vi "Configure.vi"(7 "Manual Range (1.0 V)":dbl=1.0 format="%_3g", 8 "error in (no error)":errorcluster, 9 "Manual Resolution (0: 3.5 digits)":enum16{"3.5", "4.5", "5.5", "6.5"}(ring), 10 "Function (0: DC Volts)":u16(ring) items=["DC Volts", "AC Volts"], 11 "VISA resource name":refnum<visa-resource-name>) -> (0 "error out":errorcluster, 3 "VISA resource name out":refnum<visa-resource-name>)   [LabVIEW 2019, in "K2002.lvlib"]
uses:
  K2002.lvlib
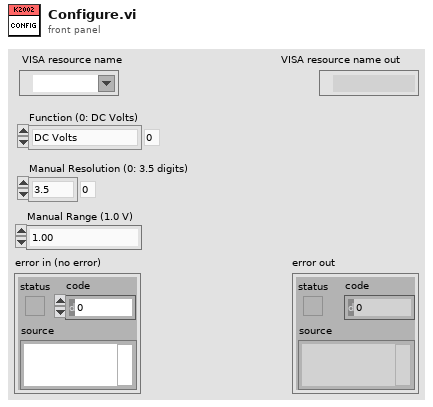
[diagram p1: front panel]
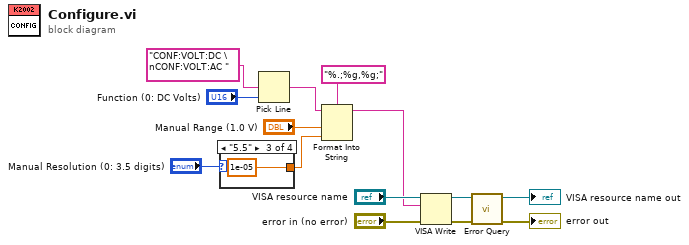
[diagram p0: block diagram]
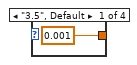
[diagram p2: hidden frame]
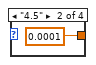
[diagram p3: hidden frame]
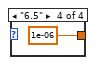
[diagram p4: hidden frame]
diagram:
  n1 = case shown="\"5.5\"" "Manual Resolution (0: 3.5 digits)" {
    tunnel: [0.001 0.0001 1e-05 1e-06] -> w1
    frame "3.5", Default {
    }
    frame "4.5" {
    }
    frame "5.5" {
    }
    frame "6.5" {
    }
  }
  n2 = Pick Line(multi-line string="CONF:VOLT:DC \nCONF:VOLT:AC " ("Function"), line index="Function (0: DC Volts)") -> (output string=w5:string)  [unwired: 1 in]
  n3 = Format Into String(format string="%.;%g,%g;", initial string=w5, "Manual Range (1.0 V)", w1) -> (resulting string=w3:string)  [unwired: 1 in, 1 out]
  n4 = VISA Write(VISA resource name="VISA resource name", write buffer=w3, error in (no error)="error in (no error)") -> (VISA resource name out=w9:refnum<visa-resource-name>, error out=w8:errorcluster)  [unwired: 1 out]
  n5 = call "Error Query.vi"("error in (no error)"=w8, "VISA resource name"=w9) -> ("error out"=→"error out":errorcluster, "VISA resource name out"=→"VISA resource name out":refnum<visa-resource-name>)  [unwired: 6 in, 2 out]
